vi "simx Get UI Slider.vi"(6 "operationMode":i32, 7 "position":i32, 8 "error in (no error)":errorcluster, 9 "uiButtonID":i32, 10 "uiHandle":i32, 11 "clientID":i32) -> (0 "error out":errorcluster, 3 "function return":i32, 5 "position out":i32)   [LabVIEW 2019, in "PXL_V-REP.lvlib"]
doc: "EXTAPI_DLLEXPORT simxInt simxGetUISlider(simxInt clientID,simxInt uiHandle,simxInt uiButtonID,simxInt* position,simxInt operationMode);"
uses:
  PXL_V-REP.lvlib
  <userlib>/V-REP/remoteApi.dll
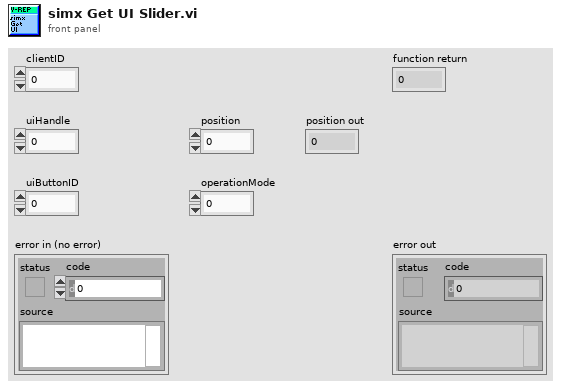
[diagram p1: front panel]
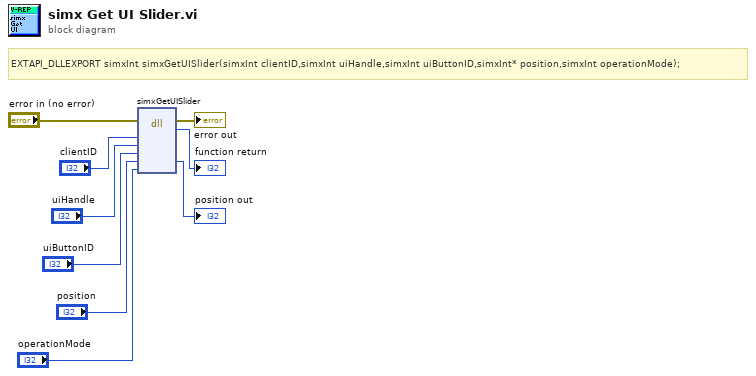
[diagram p0: block diagram]
diagram:
  # "EXTAPI_DLLEXPORT simxInt simxGetUISlider(simxInt clientID,simxInt uiHandle,simxInt uiButtonID,simxInt* position,simxInt operationMode);"
  n1 = dll-call lib="C:/Program Files (x86)/National Instruments/LabVIEW 2019/user.lib/V-REP/remoteApi.*" fn="simxGetUISlider"(error in="error in (no error)", "clientID"="clientID", "uiHandle"="uiHandle", "uiButtonID"="uiButtonID", "position"="position", "operationMode"="operationMode") -> (error out=→"error out":errorcluster, →"function return":i32, "position"=→"position out":i32)  [unwired: 6 in, 1 out]
